vi "squarecontrol_module.vi"() -> (2 "modules out":cluster{"enabled":bool[], "placing":i32[]})   [LabVIEW 2014]
panel:
  in  "reset":bool
  out "arr_found":bool[](array[boolean])
  in  "modules in":cluster{"enabled":bool[], "placing":i32[]}
  in  "finish":bool
  out "arr_locations":i32[](array[numeric])
  out "arr_bool":bool[](array[boolean])
  out "64":bool
  out "63":bool
  out "62":bool
  out "61":bool
  out "60":bool
  out "59":bool
  out "58":bool
  out "57":bool
  out "56":bool
  out "55":bool
  out "54":bool
  out "53":bool
  out "52":bool
  out "51":bool
  out "50":bool
  out "49":bool
  out "48":bool
  out "47":bool
  out "46":bool
  out "45":bool
  out "44":bool
  out "43":bool
  out "42":bool
  out "41":bool
  out "40":bool
  out "39":bool
  out "38":bool
  out "37":bool
  out "36":bool
  out "35":bool
  out "34":bool
  out "33":bool
  out "32":bool
  out "31":bool
  out "30":bool
  out "29":bool
  out "28":bool
  out "27":bool
  out "26":bool
  out "25":bool
  out "24":bool
  out "23":bool
  out "22":bool
  out "21":bool
  out "20":bool
  out "19":bool
  out "18":bool
  out "17":bool
  out "16":bool
  out "15":bool
  out "14":bool
  out "13":bool
  out "12":bool
  out "11":bool
  out "10":bool
  out "9":bool
  out "8":bool
  out "7":bool
  out "6":bool
  out "5":bool
  out "4":bool
  out "3":bool
  out "2":bool
  out "1":bool
  # "0"
  # "1"
  # "2"
  # "3"
  # "0"
  # "1"
  # "2"
  # "3"
  # "4"
  # "5"
  # "6"
  # "7"
  # "8"
  # "9"
  # "10"
  # "11"
  # "12"
  # "13"
  # "14"
  # "15"
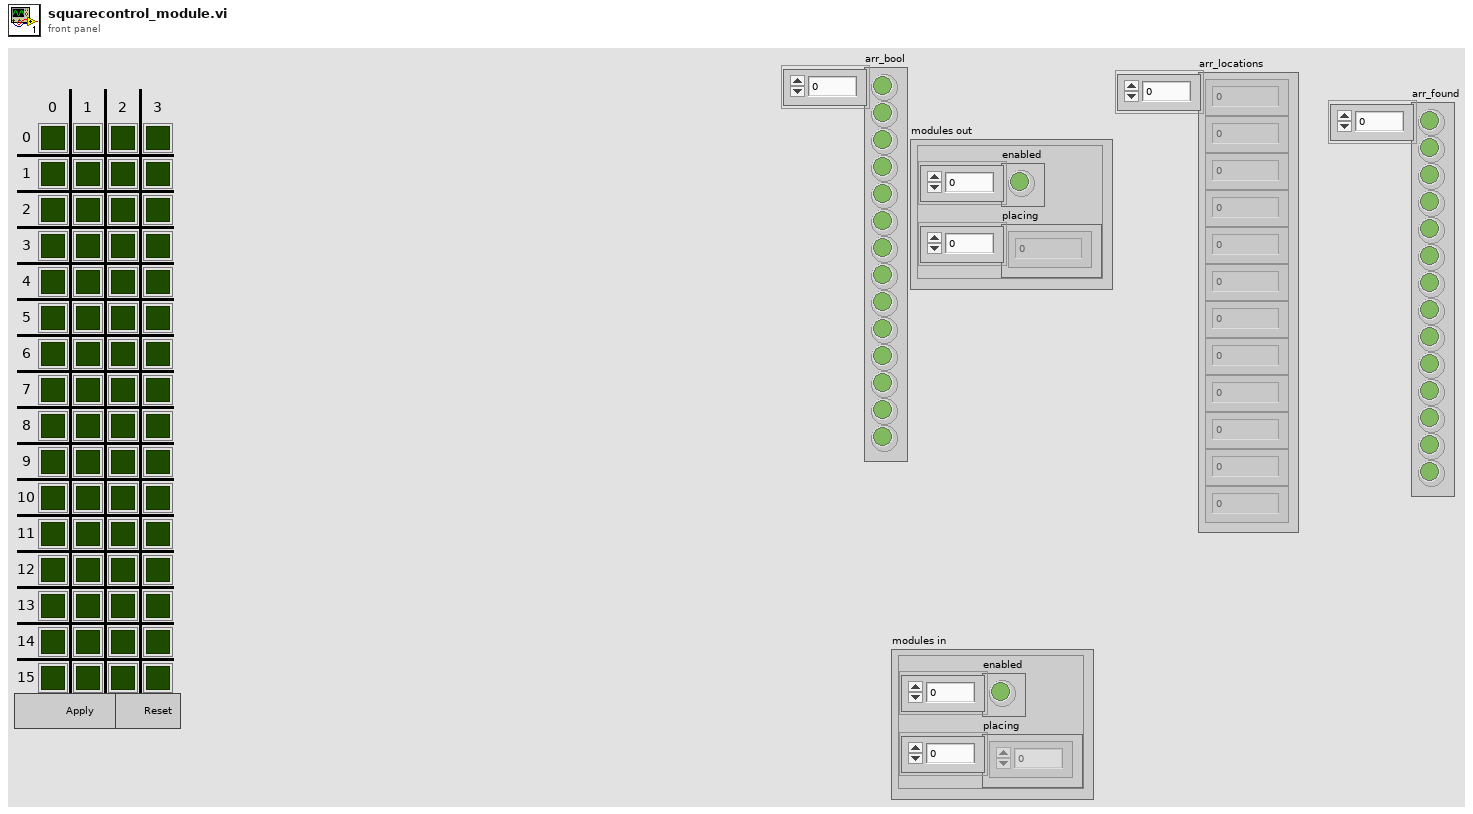
[diagram p1: front panel]
types:
  T1 = cluster{"Numeric Control":u32, "Numeric Control":u32}[]
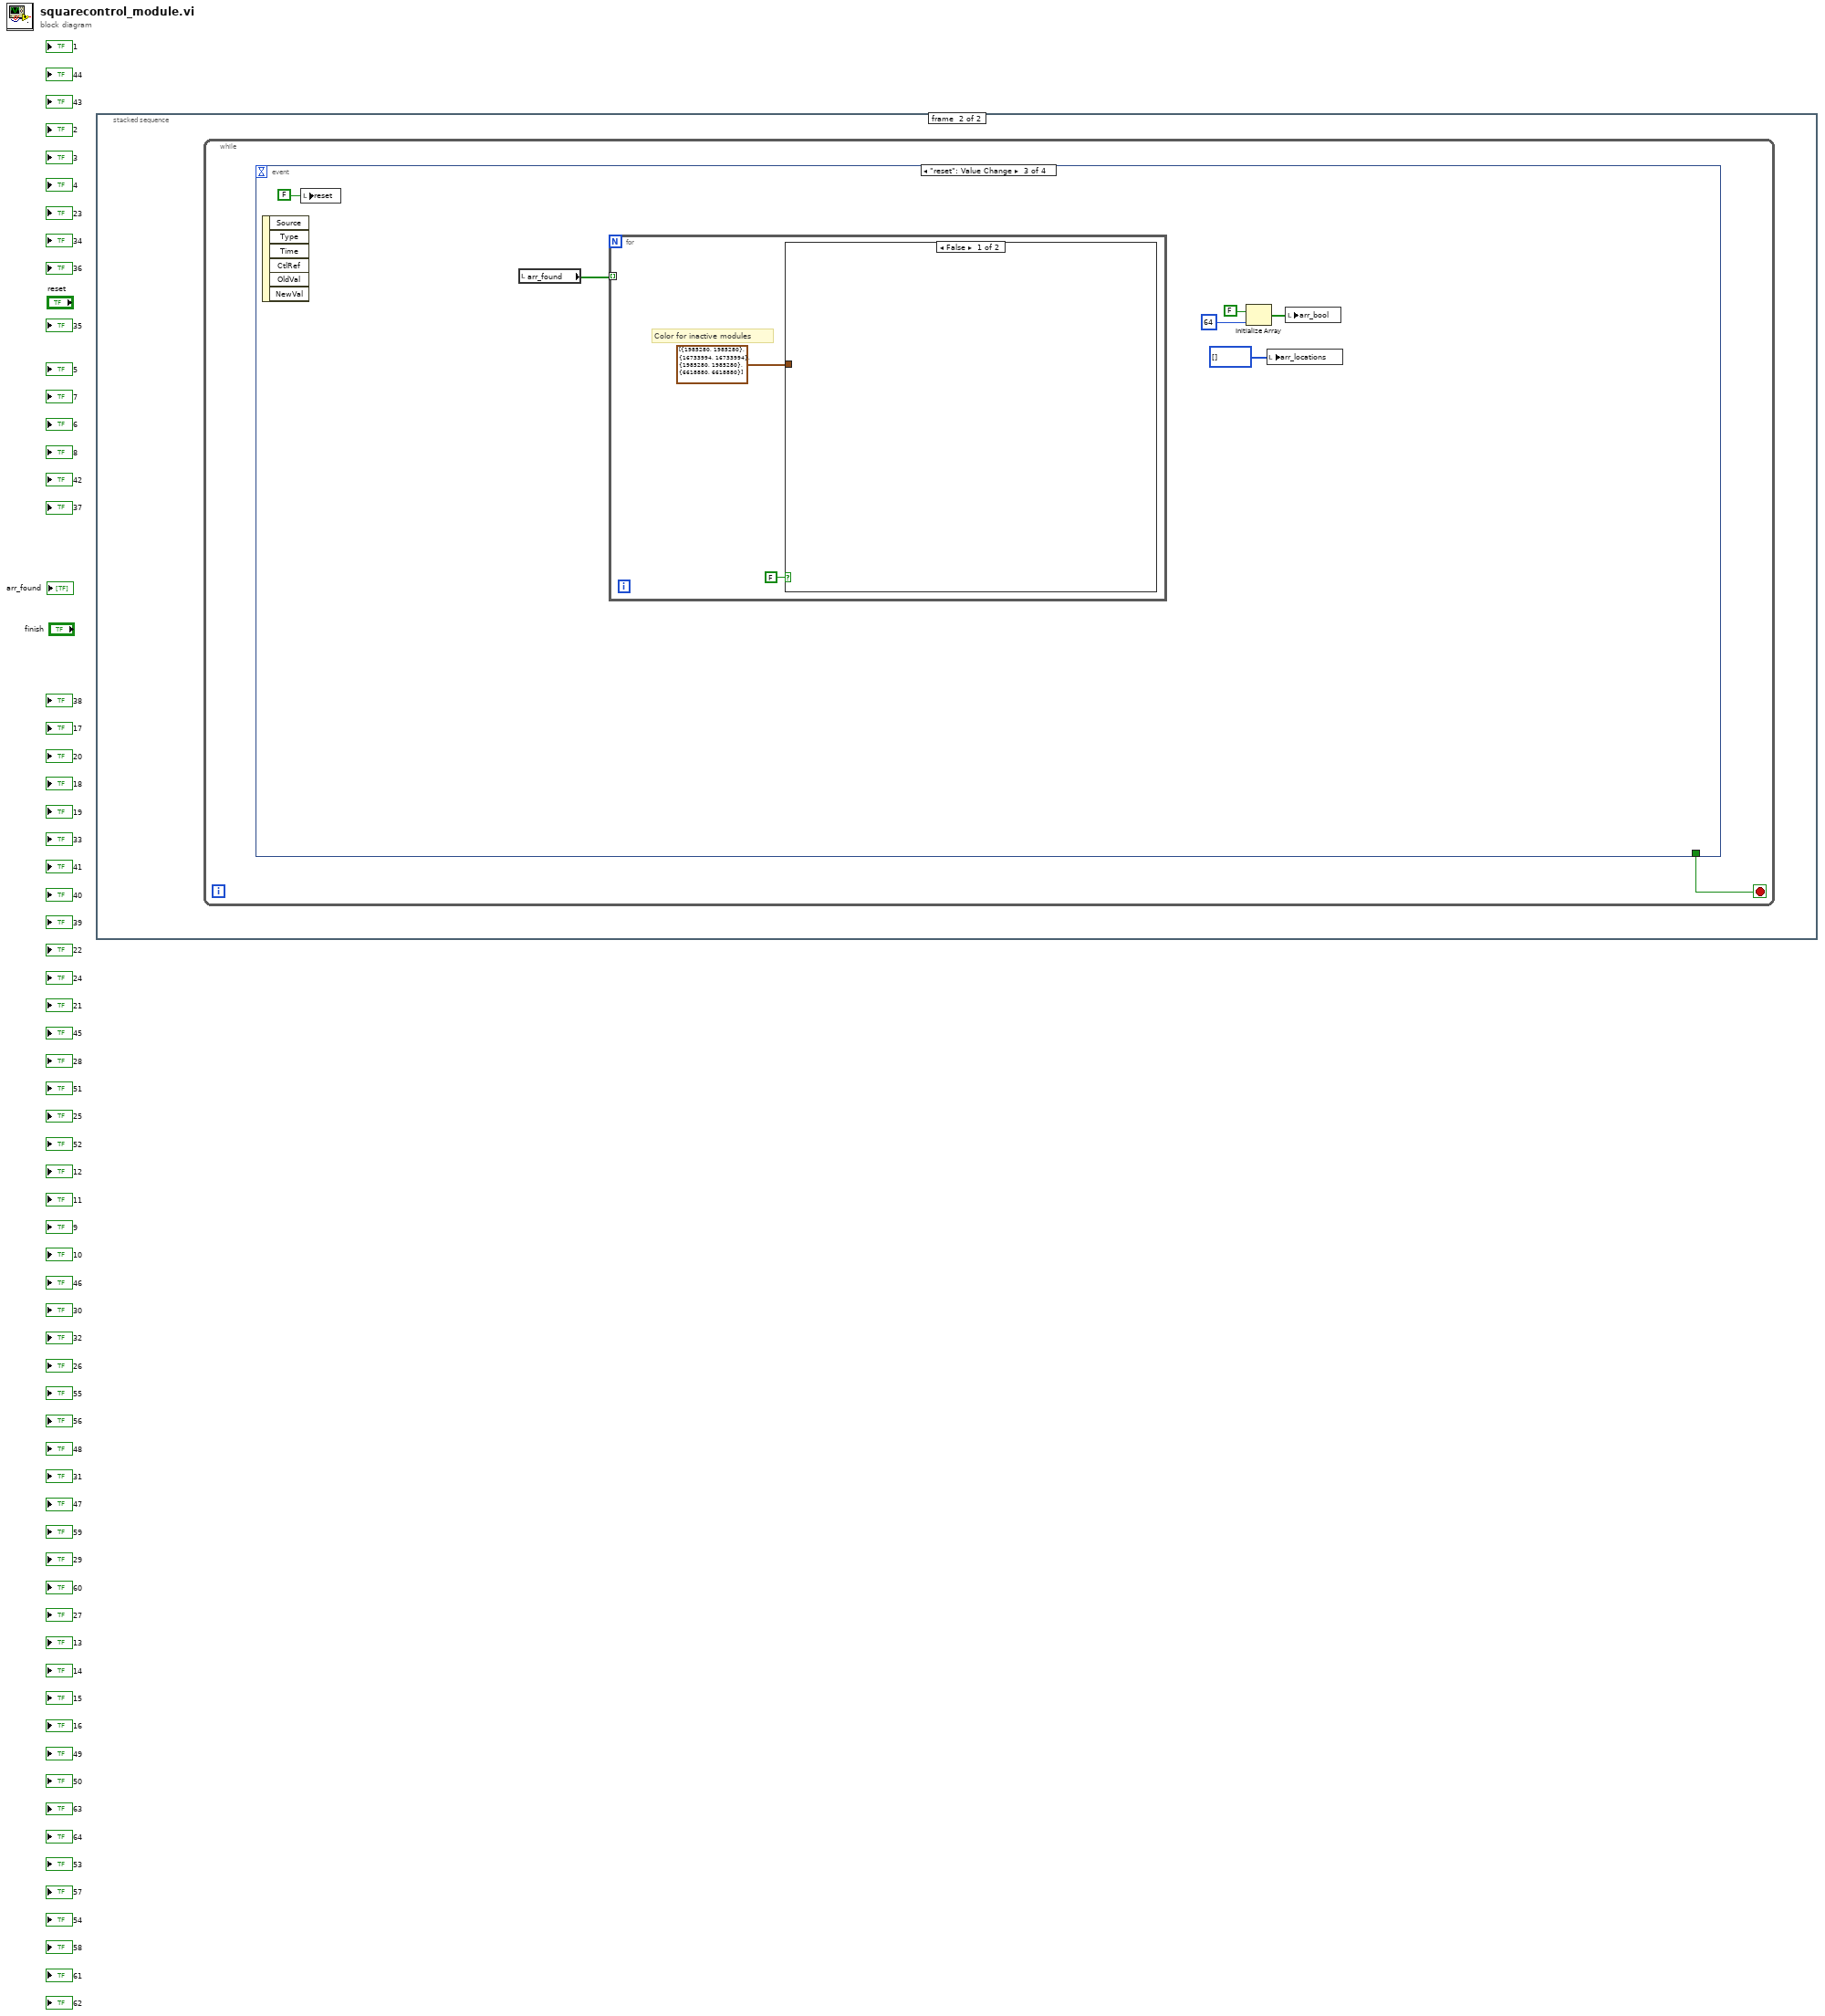
[diagram p0: block diagram]
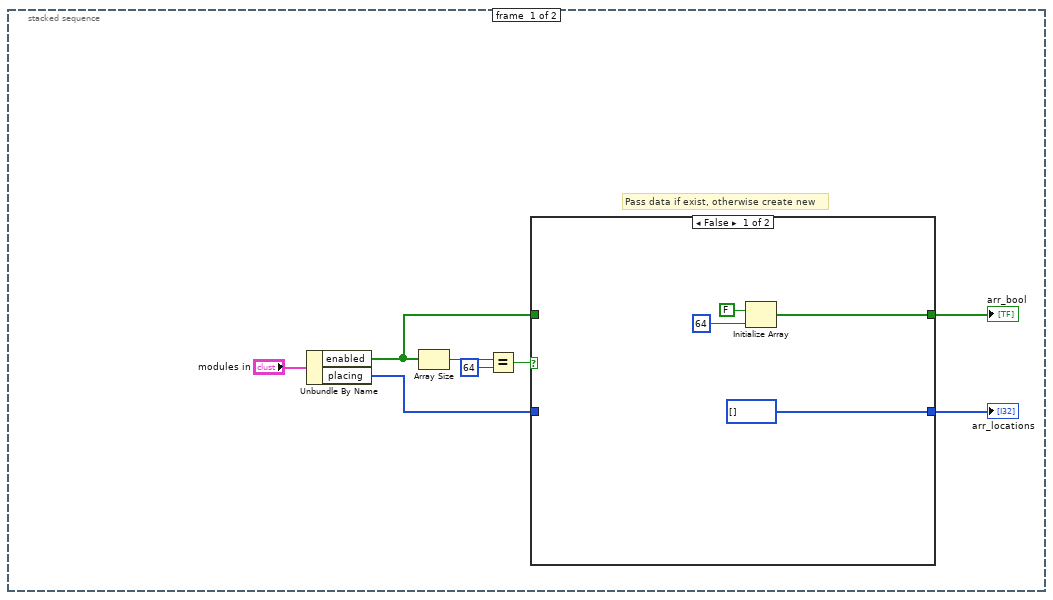
[diagram p2: hidden frame]
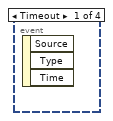
[diagram p4: hidden frame]
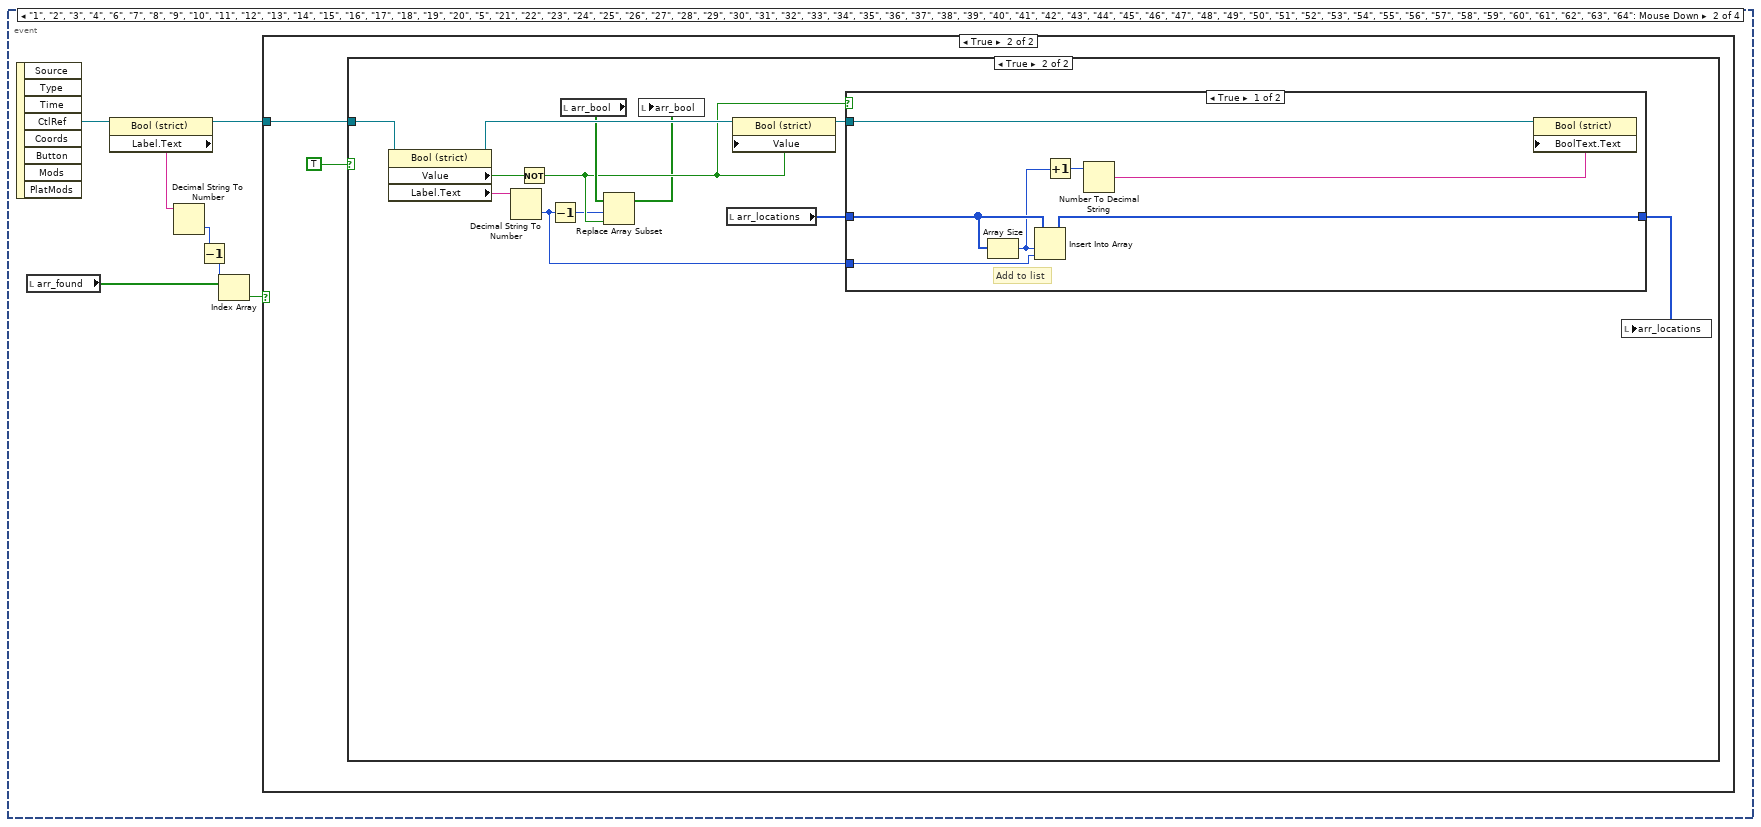
[diagram p5: hidden frame]
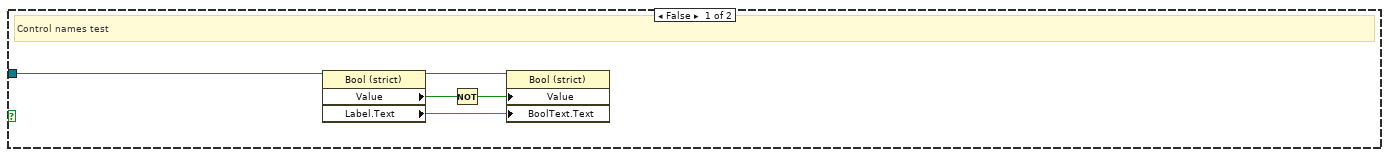
[diagram p7: hidden frame]
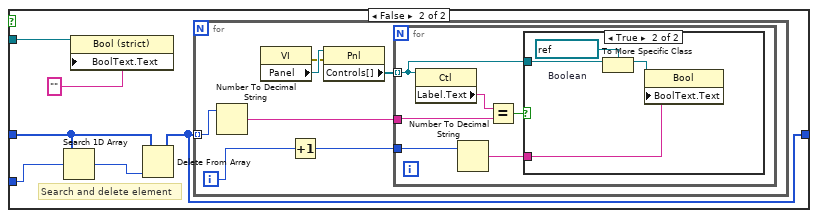
[diagram p8: hidden frame]
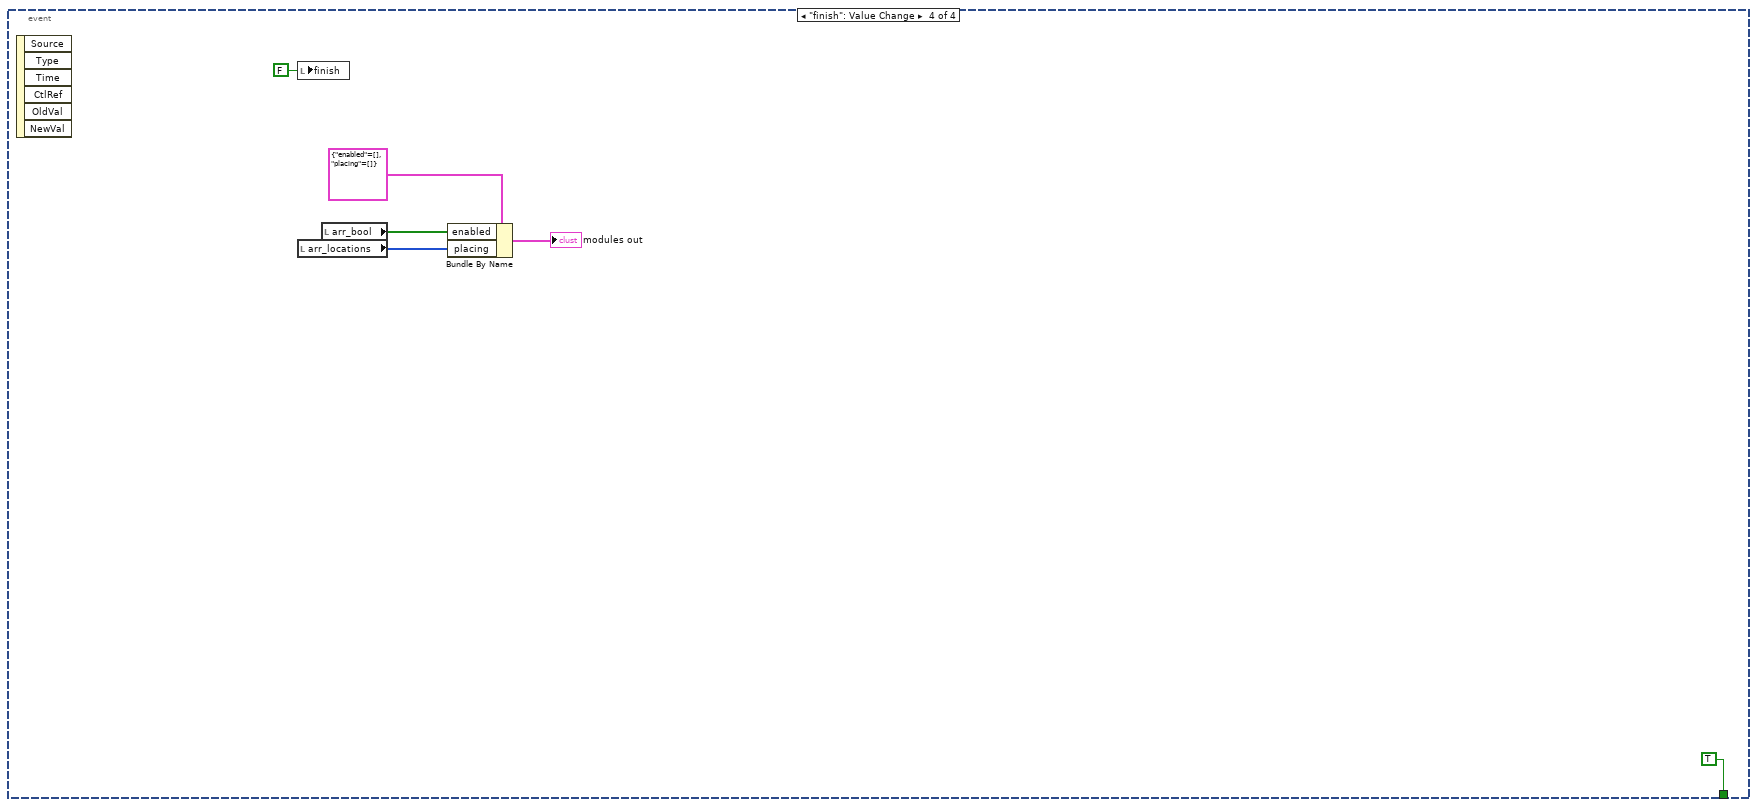
[diagram p11: hidden frame]
diagram:
  n1 = stacked-sequence {
    frame #0 {
      # "Pass data if exist, otherwise create new"
      n2 = Unbundle By Name("modules in") -> ("enabled"=w4:bool[], "placing"=w3:i32[])
      n3 = Array Size(array=w4) -> (size(s)=w7:i32)
      n4 = Equal?(x=w7, y=64) -> (x = y?=w5:bool)
      n5 = case shown="False" w5 {
        tunnel: w4 -> [_ w13]
        tunnel: w3 -> [_ w14]
        tunnel: [i32[] [] w14] -> w2
        tunnel: [w9 w13] -> w1
        frame False {
          n6 = Initialize Array(FALSE, 64 ("dimension size")) -> (w9:bool[])
        }
        frame True {
        }
      }
      "arr_bool" <- w1
      "arr_locations" <- w2
    }
    frame #1 {
      n7 = while {
        stop <- w15 stop-if-true
        n8 = event shown="[2] \"reset\": Value Change" {
          selector: _ -> [_ _ _ _]
          dyn-events: _ -> [_ _ _ _]
          timeout: _ -> [_ _ _ _]
          tunnel: [_ _ _ TRUE] -> w15
          event Timeout {
            n9 = event-data() -> ()  [unwired: 1 in, 3 out]
          }
          event "1", "2", "3", "4", "6", "7", "8", "9", "10", "11", "12", "13", "14", "15", "16", "17", "18", "19", "20", "5", "21", "22", "23", "24", "25", "26", "27", "28", "29", "30", "31", "32", "33", "34", "35", "36", "37", "38", "39", "40", "41", "42", "43", "44", "45", "46", "47", "48", "49", "50", "51", "52", "53", "54", "55", "56", "57", "58", "59", "60", "61", "62", "63", "64": Mouse Down {
            n10 = event-data() -> ("CtlRef"=w21:refnum<vi>)  [unwired: 1 in, 7 out]
            n11 = local read "arr_found"() -> (w19:bool[])
            n12 = property class="Bool (strict)"(reference=w21) -> (reference out=w22:refnum<vi>, "Label.Text"=w20:string)  [unwired: 1 in, 1 out]
            n13 = Decimal String To Number(string=w20) -> (number=w18:i32)  [unwired: 2 in, 1 out]
            n14 = Decrement(x=w18) -> (x-1=w16:i32)
            n15 = Index Array(array=w19, index=w16) -> (element=w17:bool)
            n16 = case shown="True" w17 {
              tunnel: w22 -> [_ w24]
              frame False {
              }
              frame True {
                n17 = case shown="True" TRUE {
                  tunnel: w24 -> [w29 w30]
                  frame False {
                    # "Control names test"
                    n18 = property class="Bool (strict)"(reference=w29) -> (reference out=w28:refnum<vi>, "Value"=w27:bool, "Label.Text"=w25:string)  [unwired: 1 in, 1 out]
                    n19 = Not(x=w27) -> (.not. x?=w26:bool)
                    n20 = property class="Bool (strict)"(reference=w28, "Value"=w26, "BoolText.Text"=w25) -> ()  [unwired: 1 in, 2 out]
                  }
                  frame True {
                    n21 = property class="Bool (strict)"(reference=w30) -> (reference out=w41:refnum<vi>, "Value"=w40:bool, "Label.Text"=w38:string)  [unwired: 1 in, 1 out]
                    n22 = Decimal String To Number(string=w38) -> (number=w31:i32)  [unwired: 2 in, 1 out]
                    n23 = Not(x=w40) -> (.not. x?=w36:bool)
                    n24 = Decrement(x=w31) -> (x-1=w34:i32)
                    n25 = local read "arr_bool"() -> (w37:bool[])
                    n26 = Replace Array Subset(array=w37, new element=w36, index=w34) -> (w35:bool[])
                    n27 = local write "arr_bool"(w35) -> ()
                    n28 = local read "arr_locations"() -> (w33:i32[])
                    n29 = property class="Bool (strict)"(reference=w41, "Value"=w36) -> (reference out=w39:refnum<vi>)  [unwired: 1 in, 1 out]
                    n30 = case shown="True" w36 {
                      tunnel: w39 -> [w48 w54]
                      tunnel: w33 -> [w47 w51]
                      tunnel: [w46 w49] -> w32
                      tunnel: w31 -> [w45 w52]
                      frame True {
                        # "Add to list"
                        n31 = Array Size(array=w47) -> (size(s)=w44:i32)
                        n32 = Insert Into Array(array=w47, index=w44, new element=w45) -> (w46:i32[])
                        n33 = Increment(x=w44) -> (x+1=w42:i32)
                        n34 = Number To Decimal String(number=w42) -> (decimal integer string=w43:string)  [unwired: 1 in]
                        n35 = property class="Bool (strict)"(reference=w48, "BoolText.Text"=w43) -> ()  [unwired: 1 in, 2 out]
                      }
                      frame False {
                        # "Search and delete element"
                        n36 = Search 1D Array(1D array=w51, element=w52) -> (index of element=w50:i32)  [unwired: 1 in]
                        n37 = property class="Bool (strict)"(reference=w54, "BoolText.Text"="" ("Boolean Text.Text")) -> ()  [unwired: 1 in, 2 out]
                        n38 = Delete From Array(array=w51, index=w50) -> (array with subset deleted=w49:i32[])  [unwired: 1 in, 1 out]
                        n39 = for {
                          tunnel: w49 -> [w61] mode=indexing
                          i -> [w56]
                          n40 = Number To Decimal String(number=w61) -> (decimal integer string=w57:string)  [unwired: 1 in]
                          n41 = property class="VI"() -> (error out=w59:errorcluster, "Panel"=w60:refnum<vi>)  [unwired: 2 in, 1 out]
                          n42 = Increment(x=w56) -> (x+1=w55:i32)
                          n43 = property class="Pnl"(reference=w60, error in=w59) -> ("Controls[]"=w58:refnum<vi>[])  [unwired: 2 out]
                          n44 = for {
                            tunnel: w58 -> [w62] mode=indexing
                            tunnel: w57 -> [w66]
                            tunnel: w55 -> [w64]
                            n45 = property class="Ctl"(reference=w62) -> ("Label.Text"=w67:string)  [unwired: 1 in, 2 out]
                            n46 = Number To Decimal String(number=w64) -> (decimal integer string=w63:string)  [unwired: 1 in]
                            n47 = Equal?(x=w67, y=w66) -> (x = y?=w65:bool)
                            n48 = case shown="True" w65 {
                              tunnel: w63 -> [_ w68]
                              tunnel: w62 -> [_ w71]
                              frame False {
                              }
                              frame True {
                                w70 = refnum<vi> refnum  # Boolean
                                n49 = To More Specific Class(target class=w70, reference=w71) -> (specific class reference=w69:refnum<vi>)  [unwired: 1 in, 1 out]
                                n50 = property class="Bool"(reference=w69, "BoolText.Text"=w68) -> ()  [unwired: 1 in, 2 out]
                              }
                            }
                          }
                        }
                      }
                    }
                    n51 = local write "arr_locations"(w32) -> ()
                  }
                }
              }
            }
          }
          event "reset": Value Change {
            n52 = event-data() -> ()  [unwired: 1 in, 6 out]
            n53 = local write "reset"(FALSE) -> ()
            n54 = local read "arr_found"() -> (w72:bool[])
            n55 = for {
              tunnel: w72 -> [_] mode=indexing
              # "Color for inactive modules"
              n56 = case shown="False" FALSE {
                tunnel: T1 [{"Numeric Control"=1985280, "Numeric Control"=1985280}, {"Numeric Control"=16733994, "Numeric Control"=16733994}, {"Numeric Control"=1985280, "Numeric Control"=1985280}, {"Numeric Control"=6618880, "Numeric Control"=6618880}] ("Colors [4]") -> [_ _]
                frame False {
                }
                frame True {
                }
              }
            }
            n57 = Initialize Array(FALSE, 64 ("dimension size")) -> (w74:bool[])
            n58 = local write "arr_locations"(i32[] []) -> ()
            n59 = local write "arr_bool"(w74) -> ()
          }
          event "finish": Value Change {
            n60 = event-data() -> ()  [unwired: 1 in, 6 out]
            n61 = local write "finish"(FALSE ("finish")) -> ()
            n62 = local read "arr_locations"() -> (w82:i32[])
            n63 = local read "arr_bool"() -> (w83:bool[])
            n64 = Bundle By Name(cluster=cluster{"enabled":bool[], "placing":i32[]} {"enabled"=[], "placing"=[]}, "enabled"=w83, "placing"=w82) -> (→"modules out":cluster{"enabled":bool[], "placing":i32[]})
          }
        }
      }
    }
  }
